vi "List Script.vi"(8 "error in (no error)":errorcluster, 10 "Script Variable":string, 11 "VISA resource name":refnum<visa-resource-name>) -> (0 "error out":errorcluster, 2 "Script List":string[](array[string]), 3 "VISA resource name out":refnum<visa-resource-name>)   [LabVIEW 2019, in "Keithley 2600 Series.lvlib"]
doc: "Generates a script listing."
uses:
  Keithley 2600 Series.lvlib
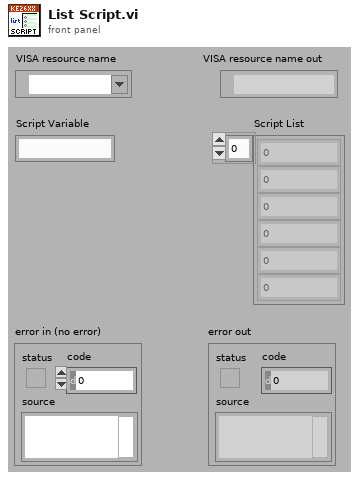
[diagram p1: front panel]
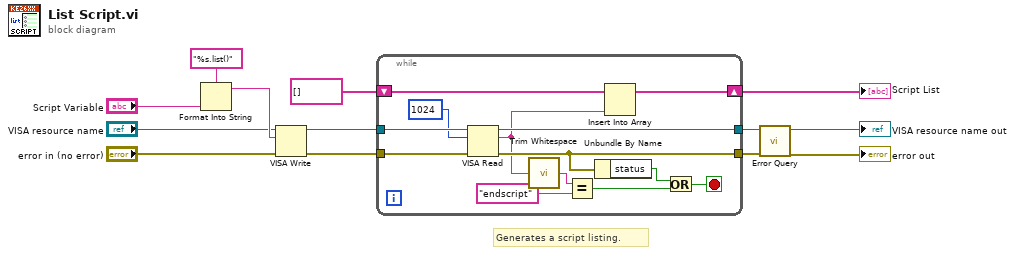
[diagram p0: block diagram]
diagram:
  # "Generates a script listing."
  n1 = Format Into String(format string="%s.list()", "Script Variable") -> (resulting string=w11:string)  [unwired: 2 in, 1 out]
  n2 = VISA Write(VISA resource name="VISA resource name", write buffer=w11, error in (no error)="error in (no error)") -> (VISA resource name out=w6:refnum<visa-resource-name>, error out=w5:errorcluster)  [unwired: 1 out]
  n3 = while {
    tunnel: w6 -> [w26]
    tunnel: w5 -> [w25]
    tunnel: [w24] -> w2
    tunnel: [w19] -> w1
    shift-right: [w20] -> w3
    shift-left: string[] [] ("array") -> [w21]
    stop <- w18 stop-if-true
    n4 = VISA Read(VISA resource name=w26, byte count=u32 1024, error in (no error)=w25) -> (VISA resource name out=w24:refnum<visa-resource-name>, read buffer=w14:string, error out=w19:errorcluster)  [unwired: 1 out]
    n5 = call <vilib>:"Trim Whitespace.vi"("string"=w14) -> ("trimmed string"=w15:string)  [unwired: 1 in]
    n6 = Equal?(x=w15, y="endscript") -> (x = y?=w17:bool)
    n7 = Unbundle By Name(w19) -> ("status"=w16:bool)
    n8 = Insert Into Array(array=w21, new element=w14) -> (w20:string[])  [unwired: 1 in]
    n9 = Or(x=w16, y=w17) -> (x .or. y?=w18:bool)
  }
  "Script List" <- w3
  n10 = call "Error Query.vi"("error in (no error)"=w1, "VISA resource name"=w2) -> ("error out"=→"error out":errorcluster, "VISA resource name out"=→"VISA resource name out":refnum<visa-resource-name>)  [unwired: 6 in, 2 out]
